vi "Shooter.vi"(8 "error in (no error)":errorcluster) -> ()   [LabVIEW 2014]
uses:
  <vilib>/Rock Robotics/WPI/Relay/WPI_RelayValue.ctl
  Shooter State Enum.ctl
  Robot Global Data.vi
  <vilib>/Rock Robotics/Network Tables/SD Write Number.vi
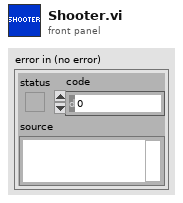
[diagram p1: front panel]
types:
  T1 = typedef "Shooter State Enum.ctl" = enum16{"Ready", "Fired", "DrawingToReady"}
  T2 = typedef "WPI_MotorControlDeviceRef.ctl" = cluster{"DeviceStatus":errorcluster, "Type":enum16{"PWM", "CAN"}, "PWM":cluster{"Digital Module":T3, "PWM Channel":T4, "DeadBand":T5}, "CAN":cluster{"Device Number":u8, "Control Mode":T6, "Semaphore":T7, "Max Vout":dbl}, "Invert":bool, "TransformRef":T8, "InvTransformRef":T8}
  T3 = typedef "FPGA_TypedefDigitalModule.ctl" = enum16{"Digital Module 1", "Digital Module 2"}
  T4 = typedef "FPGA_DIOPWMChannel.ctl" = enum8{"PWM 1", "PWM 2", "PWM 3", "PWM 4", "PWM 5", "PWM 6", "PWM 7", "PWM 8", "PWM 9", "PWM 10", "Invalid"}
  T5 = typedef "WPI_PWMDeadband.ctl" = cluster{"Name":string, "maxPositivePwm":i32, "minPositivePwm":i32, "centerPwm":i32, "maxNegativePwm":i32, "minNegativePwm":i32, "angularRange":u16}
  T6 = typedef "WPI_CANJaguar_ControlMode.ctl" = enum8{"Percent VBus", "Current", "Speed", "Position", "Voltage"}
  T7 = typedef "Semaphore RefNum" = refnum<k1>
  T8 = typedef "WPI_PWMTransform_ConPane.ctl" = refnum<vi>
  T9 = typedef "WPI_RelayDevRef.ctl" = cluster{"DevStatus":errorcluster, "Relay Channel":T10, "Digital Module":T3, "Relay Direction":T11}
  T10 = typedef "FPGA_DIORelayChannel.ctl" = enum8{"Relay 1", "Relay 2", "Relay 3", "Relay 4", "Relay 5", "Relay 6", "Relay 7", "Relay 8", "Invalid"}
  T11 = typedef "WPI_RelayDirection.ctl" = enum16{"Both directions", "Forward only", "Reverse only"}
  T12 = typedef "WPI_RelayValue.ctl" = enum16{"Off", "On", "Forward", "Reverse"}
  T13 = typedef "User Commands typedef.ctl" = cluster{"Arm Command":T14, "Shooter Commands":T16, "Drive Commands":T17}
  T14 = typedef "Arm control typedef.ctl" = cluster{"Arm up/dwn":dbl, "Arm Capture":bool, "Arm Pass":bool, "Arm Positions":T15, "Arm Manual Override":bool}
  T15 = typedef "Arm Postions Enum Typedef.ctl" = enum16{"Arm Pick-up", "Idle", "Arm Shoot", "Arm Truss", "Manual"}
  T16 = typedef "Shooter Commands Typedef.ctl" = cluster{"Shooter Fire":bool, "Shooter Draw":bool}
  T17 = typedef "Drive Commands Typedef.ctl" = cluster{"Drive L/R":dbl, "Drive Fwd/Rev":dbl}
  T18 = typedef "Robot Info Typedef.ctl" = cluster{"Arm Info":T19, "Shooter Info":T20}
  T19 = typedef "Arm Info Typedef.ctl" = cluster{"Current Arm Position":dbl, "Arm Bottom Limit Switch":bool, "Arm Top Limit Switch":bool}
  T20 = typedef "Shooter Info Typedef.ctl" = cluster{"Shooter At Full":bool}
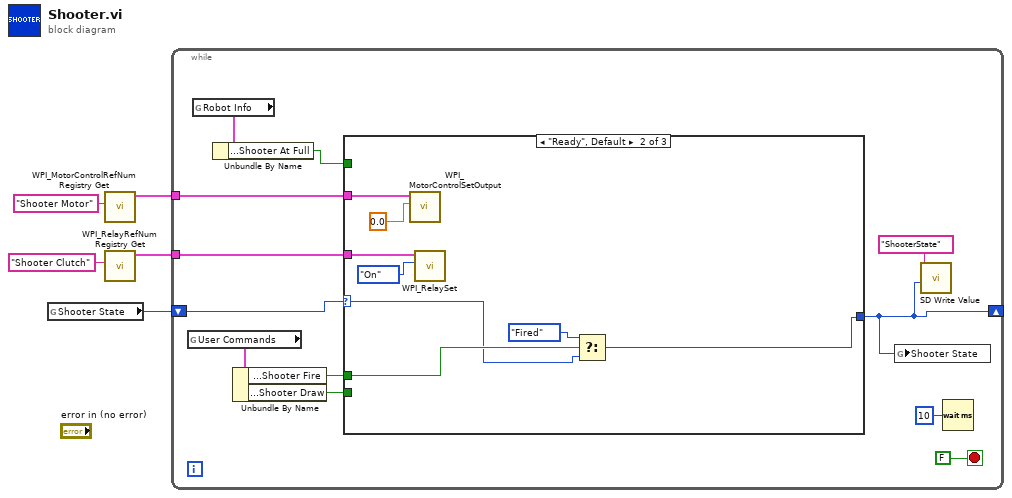
[diagram p0: block diagram]
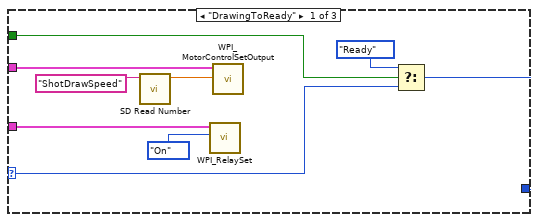
[diagram p2: hidden frame]
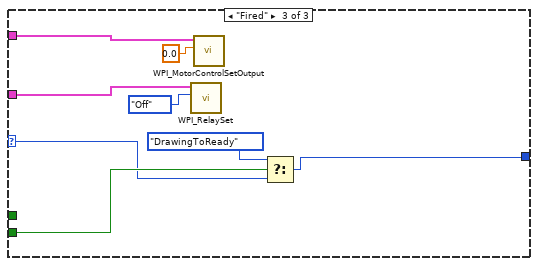
[diagram p3: hidden frame]
diagram:
  n1 = global read "Robot Global Data.vi" "Shooter State"() -> (w5:T1)
  n2 = call <vilib>:"WPI_MotorControlRefNum Registry Get.vi"("refnum name"="Shooter Motor") -> ("MotorControlDevRef"=w2:T2)  [unwired: 9 in, 1 out]
  n3 = call <vilib>:"WPI_RelayRefNum Registry Get.vi"("refnum name"="Shooter Clutch") -> ("RelayDevRef"=w1:T9)  [unwired: 9 in, 1 out]
  n4 = while {
    shift-right: [w9] -> _
    shift-left: w5 -> [w16]
    tunnel: w2 -> [w15]
    tunnel: w1 -> [w14]
    stop <- FALSE stop-if-true
    n5 = global read "Robot Global Data.vi" "User Commands"() -> (w13:T13)
    n6 = global read "Robot Global Data.vi" "Robot Info"() -> (w7:T18)
    n7 = Unbundle By Name(w7) -> ("Shooter Info.Shooter At Full"=w6:bool)
    n8 = Unbundle By Name(w13) -> ("Shooter Commands.Shooter Fire"=w11:bool, "Shooter Commands.Shooter Draw"=w12:bool)
    n9 = case shown="\"Ready\", Default" w16 {
      selector: w16 -> [w20 w28 w37]
      tunnel: w15 -> [w24 w34 w42]
      tunnel: w14 -> [w23 w32 w40]
      tunnel: w12 -> [_ _ w38]
      tunnel: [w19 w27 w35] -> w9
      tunnel: w11 -> [_ w29 _]
      tunnel: w6 -> [w18 _ _]
      frame "DrawingToReady" {
        n10 = call <vilib>:"SD Read Number.vi"("Name"="ShotDrawSpeed") -> ("Numeric"=w22:dbl)  [unwired: 8 in, 2 out]
        n11 = call <vilib>:"WPI_RelaySet.vi"("RelayValue"=WPI_RelayValue."On", "RelayDevRef"=w23) -> ()  [unwired: 8 in, 2 out]
        n12 = call <vilib>:"WPI_MotorControlSetOutput.vi"("Output"=w22, "MotorControlDevRef"=w24) -> ()  [unwired: 7 in, 3 out]
        n13 = Select(t=Shooter_State_Enum."Ready", s=w18, f=w20) -> (s? t:f=w19:T1)
      }
      frame "Ready", Default {
        n14 = call <vilib>:"WPI_MotorControlSetOutput.vi"("Output"=0.0, "MotorControlDevRef"=w34) -> ()  [unwired: 7 in, 3 out]
        n15 = call <vilib>:"WPI_RelaySet.vi"("RelayValue"=WPI_RelayValue."On", "RelayDevRef"=w32) -> ()  [unwired: 8 in, 2 out]
        n16 = Select(t=Shooter_State_Enum."Fired", s=w29, f=w28) -> (s? t:f=w27:T1)
      }
      frame "Fired" {
        n17 = call <vilib>:"WPI_RelaySet.vi"("RelayValue"=WPI_RelayValue."Off", "RelayDevRef"=w40) -> ()  [unwired: 8 in, 2 out]
        n18 = call <vilib>:"WPI_MotorControlSetOutput.vi"("Output"=0.0, "MotorControlDevRef"=w42) -> ()  [unwired: 7 in, 3 out]
        n19 = Select(t=Shooter_State_Enum."DrawingToReady", s=w38, f=w37) -> (s? t:f=w35:T1)
      }
    }
    n20 = global write "Robot Global Data.vi" "Shooter State"(w9) -> ()
    n21 = call-poly <vilib>:"SD Write Value.vi"("Numeric"=w9, "Name"="ShooterState") -> ()  [unwired: 8 in, 2 out]
    n22 = Wait (ms)(milliseconds to wait=u32 10) -> ()  [unwired: 1 out]
  }
